vi "污染物CP编码.vi"(5 "table":string="雷达流速仪", 6 "地表水/污染源":bool, 7 "字符串":string="N", 8 "字段结束":bool=TRUE, 9 "数据类型":string(combo)="-Rtd=", 10 "污染物浓度":string, 11 "污染物编码":string) -> (3 "编码输出":string)   [LabVIEW 2016, in "数据传输系统-03.lvlib"]
panel:
  in  "设备类型":string(combo)="010200"
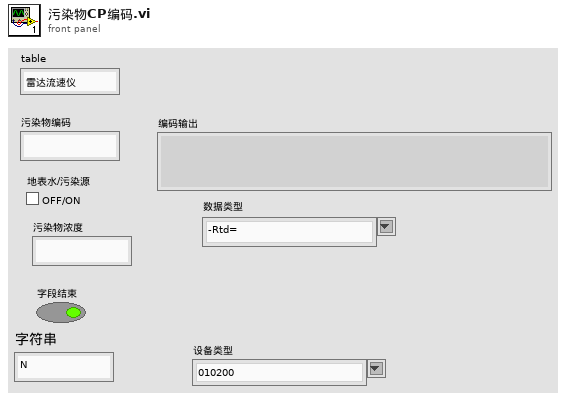
[diagram p1: front panel]
types:
  T1 = typedef "LVComboBoxStrsAndValuesArrayTypeDef.ctl" = cluster{"String":string, "Value":string}[]
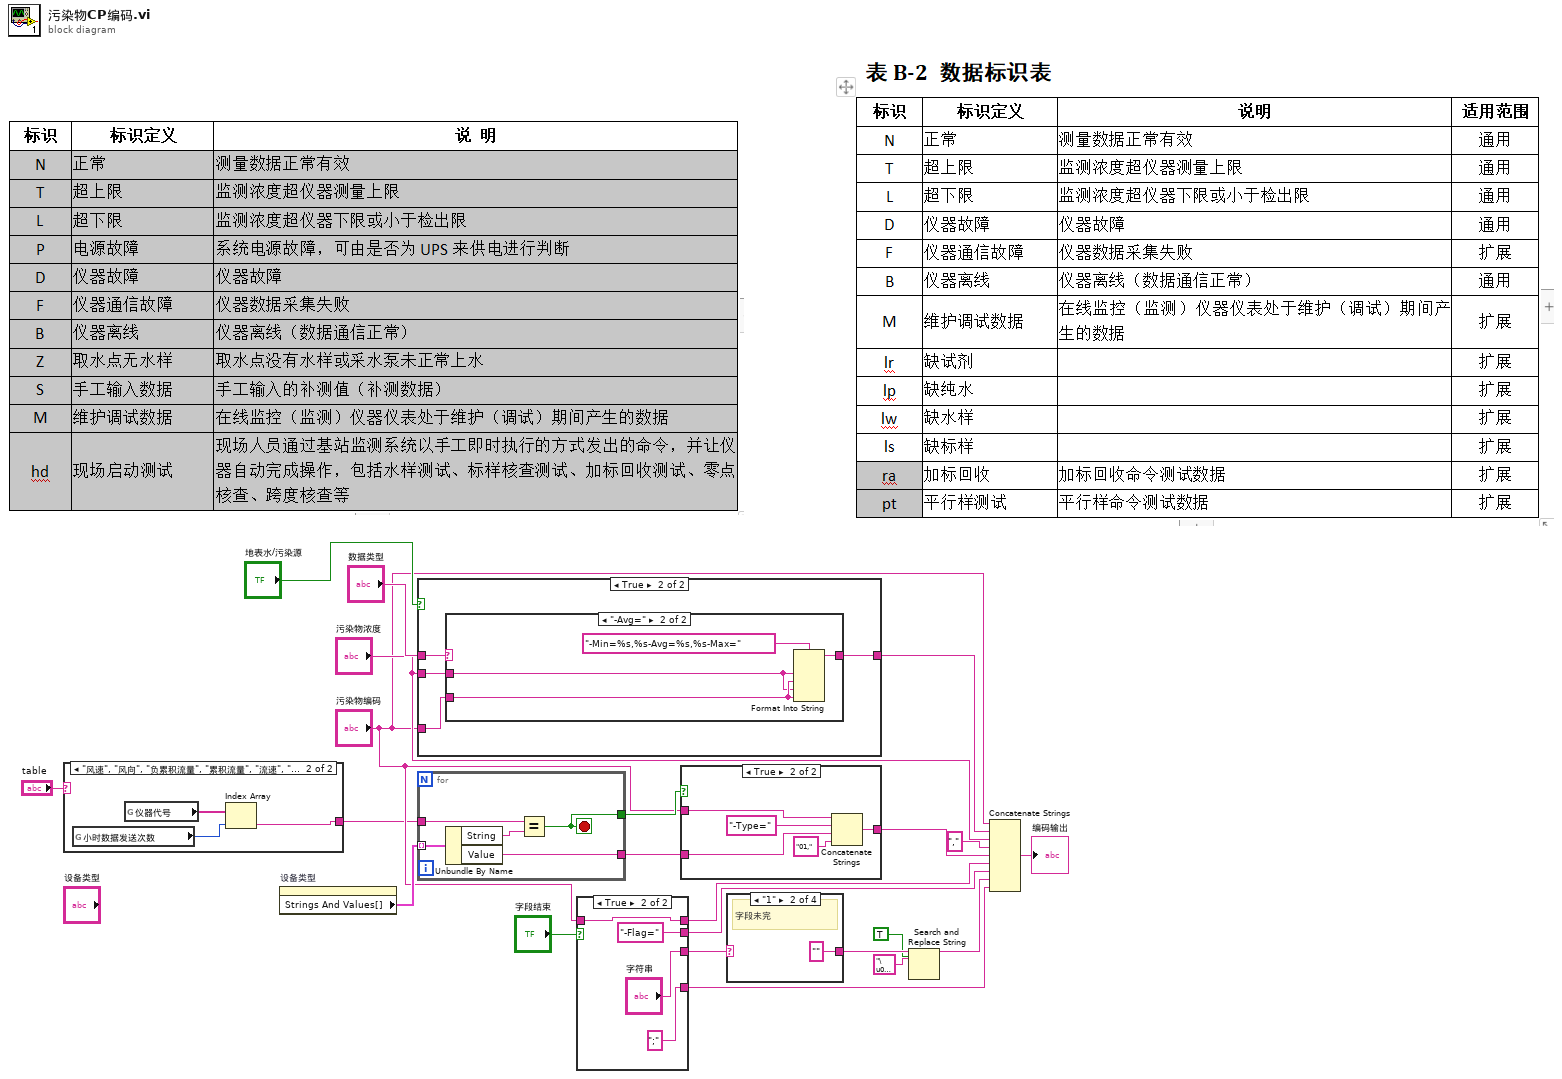
[diagram p0: block diagram]
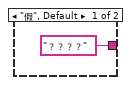
[diagram p2: hidden frame]
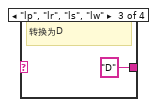
[diagram p7: hidden frame]
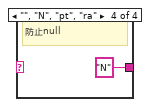
[diagram p8: hidden frame]
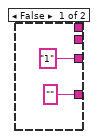
[diagram p9: hidden frame]
diagram:
  n1 = case shown="\"风速\", \"风向\", \"负累积流量\", \"累积流量\", \"流速\", \"气温\", \"气压\", \"水位\", \"瞬时流量\", \"正累积流量\"" "table" {
    tunnel: ["？？？？" w25] -> w1
    frame "假", Default {
    }
    frame "风速", "风向", "负累积流量", "累积流量", "流速", "气温", "气压", "水位", "瞬时流量", "正累积流量" {
      n2 = global read "全局 小时数据发送次数.vi" "小时数据发送次数"() -> (w24:i32)
      n3 = global read "全局 所有参数.vi" "仪器代号"() -> (w26:string[])
      n4 = Index Array(array=w26, index=w24) -> (element=w25:string)
    }
  }
  n5 = property on="设备类型" class="CmbBox"() -> ("Strings And Values[]"=w8:T1)  [unwired: 2 in, 2 out]
  n6 = case shown="True" "地表水/污染源" {
    tunnel: "数据类型" -> [w27 w31]
    tunnel: [w27 w30] -> w10
    tunnel: "污染物编码" -> [_ w29]
    tunnel: "污染物浓度" -> [_ w28]
    frame False {
    }
    frame True {
      n7 = case shown="\"-Avg=\"" w31 {
        selector: w31 -> [w32 _]
        tunnel: [w32 w33] -> w30
        tunnel: w29 -> [_ w35]
        tunnel: w28 -> [_ w34]
        frame "假", Default {
        }
        frame "-Avg=" {
          n8 = Format Into String(format string="-Min=%s,%s-Avg=%s,%s-Max=" ("格式字符串"), w34, w35, w34, w35) -> (resulting string=w33:string)  [unwired: 2 in, 1 out]
        }
      }
    }
  }
  n9 = for {
    tunnel: w8 -> [w41] mode=indexing
    tunnel: w1 -> [w39]
    tunnel: [w38] -> w6
    tunnel: [w37] -> w7
    stop <- w37 stop-if-true
    n10 = Unbundle By Name(w41) -> ("String"=w40:string, "Value"=w38:string)
    n11 = Equal?(x=w39, y=w40) -> (x = y?=w37:bool)
  }
  n12 = case shown="True" "字段结束" {
    tunnel: [_ "-Flag=" ("字符串")] -> w21
    tunnel: ["1" ("字符串") "字符串"] -> w18
    tunnel: "污染物编码" -> [_ w46]
    tunnel: [_ w46] -> w19
    tunnel: ["" ("字符串") ";" ("字符串")] -> w13
    frame False {
    }
    frame True {
    }
  }
  n13 = case shown="True" w7 {
    tunnel: w6 -> [_ w50]
    tunnel: "污染物编码" -> [_ w52]
    tunnel: [_ w48] -> w3
    frame False {
    }
    frame True {
      n14 = Concatenate Strings(w52, "-Type=" ("格式字符串"), w50, "01," ("字符串")) -> (w48:string)
    }
  }
  n15 = case shown="\"1\"" w18 {
    selector: w18 -> [w53 _ _ _]
    tunnel: [w53 "" ("字符串") "D" ("字符串") "N" ("字符串")] -> w17
    frame Default {
      # "其他透传"
    }
    frame "1" {
      # "字段未完"
    }
    frame "lp", "lr", "ls", "lw" {
      # "转换为D"
    }
    frame "", "N", "pt", "ra" {
      # "防止null"
    }
  }
  n16 = Search and Replace String(replace all?=TRUE ("替换全部？(F)"), input string=w17, search string="\u0000" ("搜索字符串")) -> (result string=w15:string)  [unwired: 5 in, 3 out]
  n17 = Concatenate Strings("污染物编码", w10, "污染物浓度", "," ("字符串"), w3, w19, w21, w15, w13) -> (→"编码输出":string)
